vi "poly_merge_errors_up.vi"(9 "sub error":errorcluster, 10 "main error":errorcluster) -> (2 "error out":errorcluster)   [LabVIEW 2015]
panel:
  # "WIP"
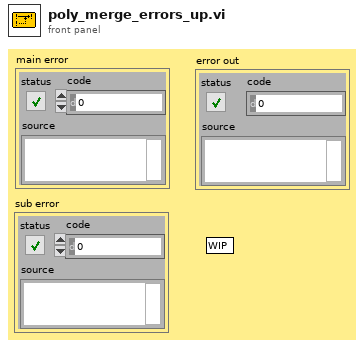
[diagram p1: front panel]
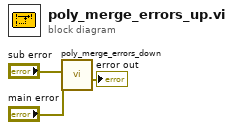
[diagram p0: block diagram]
diagram:
  n1 = call "poly_merge_errors_down.vi"("main error"="main error", "sub error"="sub error") -> ("error out"=→"error out":errorcluster)  [unwired: 9 in]
